vi "XVC_SERVER_UDP.vi"() -> ()   [LabVIEW 2017]
panel:
  out "error out":errorcluster caption="错误输出"
  out "连接的字符串":string
  out "错误输出 5":errorcluster caption="错误输出"
  out "错误输出 4":errorcluster caption="错误输出"
  out "字符串":string
  out "错误输出 3":errorcluster={"status"=TRUE, "code"=56, "source"="TCP Listen.vi:7210001->XVC_SERVER_UDP.vi中的等待TCP侦听器"} caption="错误输出"
  out "错误输出 2":errorcluster={"status"=TRUE, "code"=1, "source"="XVC_SERVER_UDP.vi中的关闭TCP连接"} caption="错误输出"
  out "错误输出":errorcluster
  out "x+1":u32
  in  "data out 5":string="shift:\u0005\u0000\u0000\u0000ÿ\u0000"
  out "received string 2":string
  in  "address":string="192.168.10.20"
  out "received string":string
  out "data out 3":string
  in  "data out 4":string="shift:\u0005\u0000\u0000\u0000ÿ\u0000"
  out "data out 2":string
  out "x != 0?":bool
  in  "Client Closed":string="The client VI closed the connection."
  in  "Stop":bool
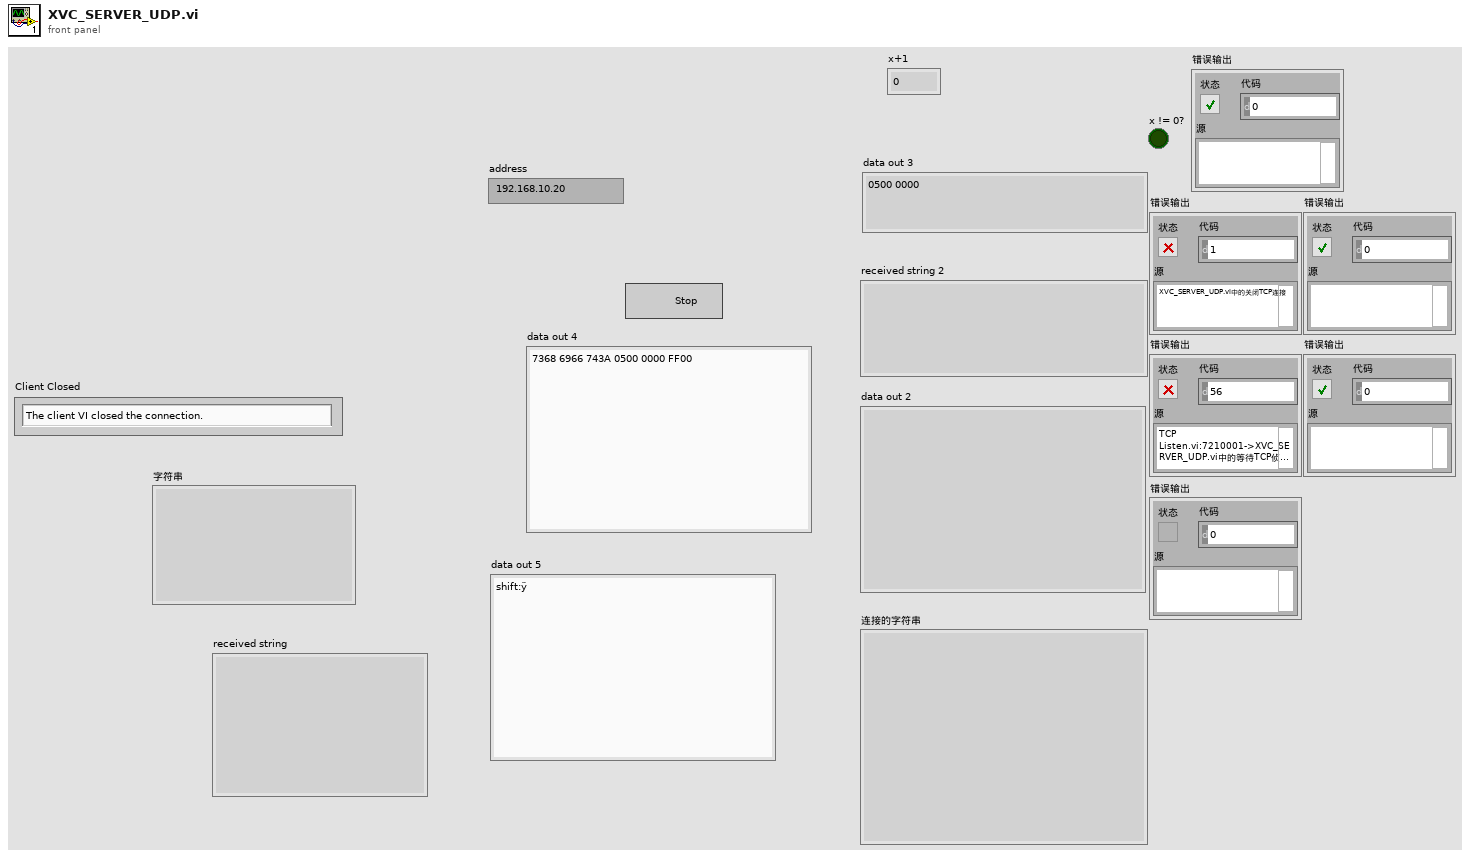
[diagram p1: front panel]
types:
  T1 = enum16{"Standard", "Buffered", "CRLF", "Immediate"}
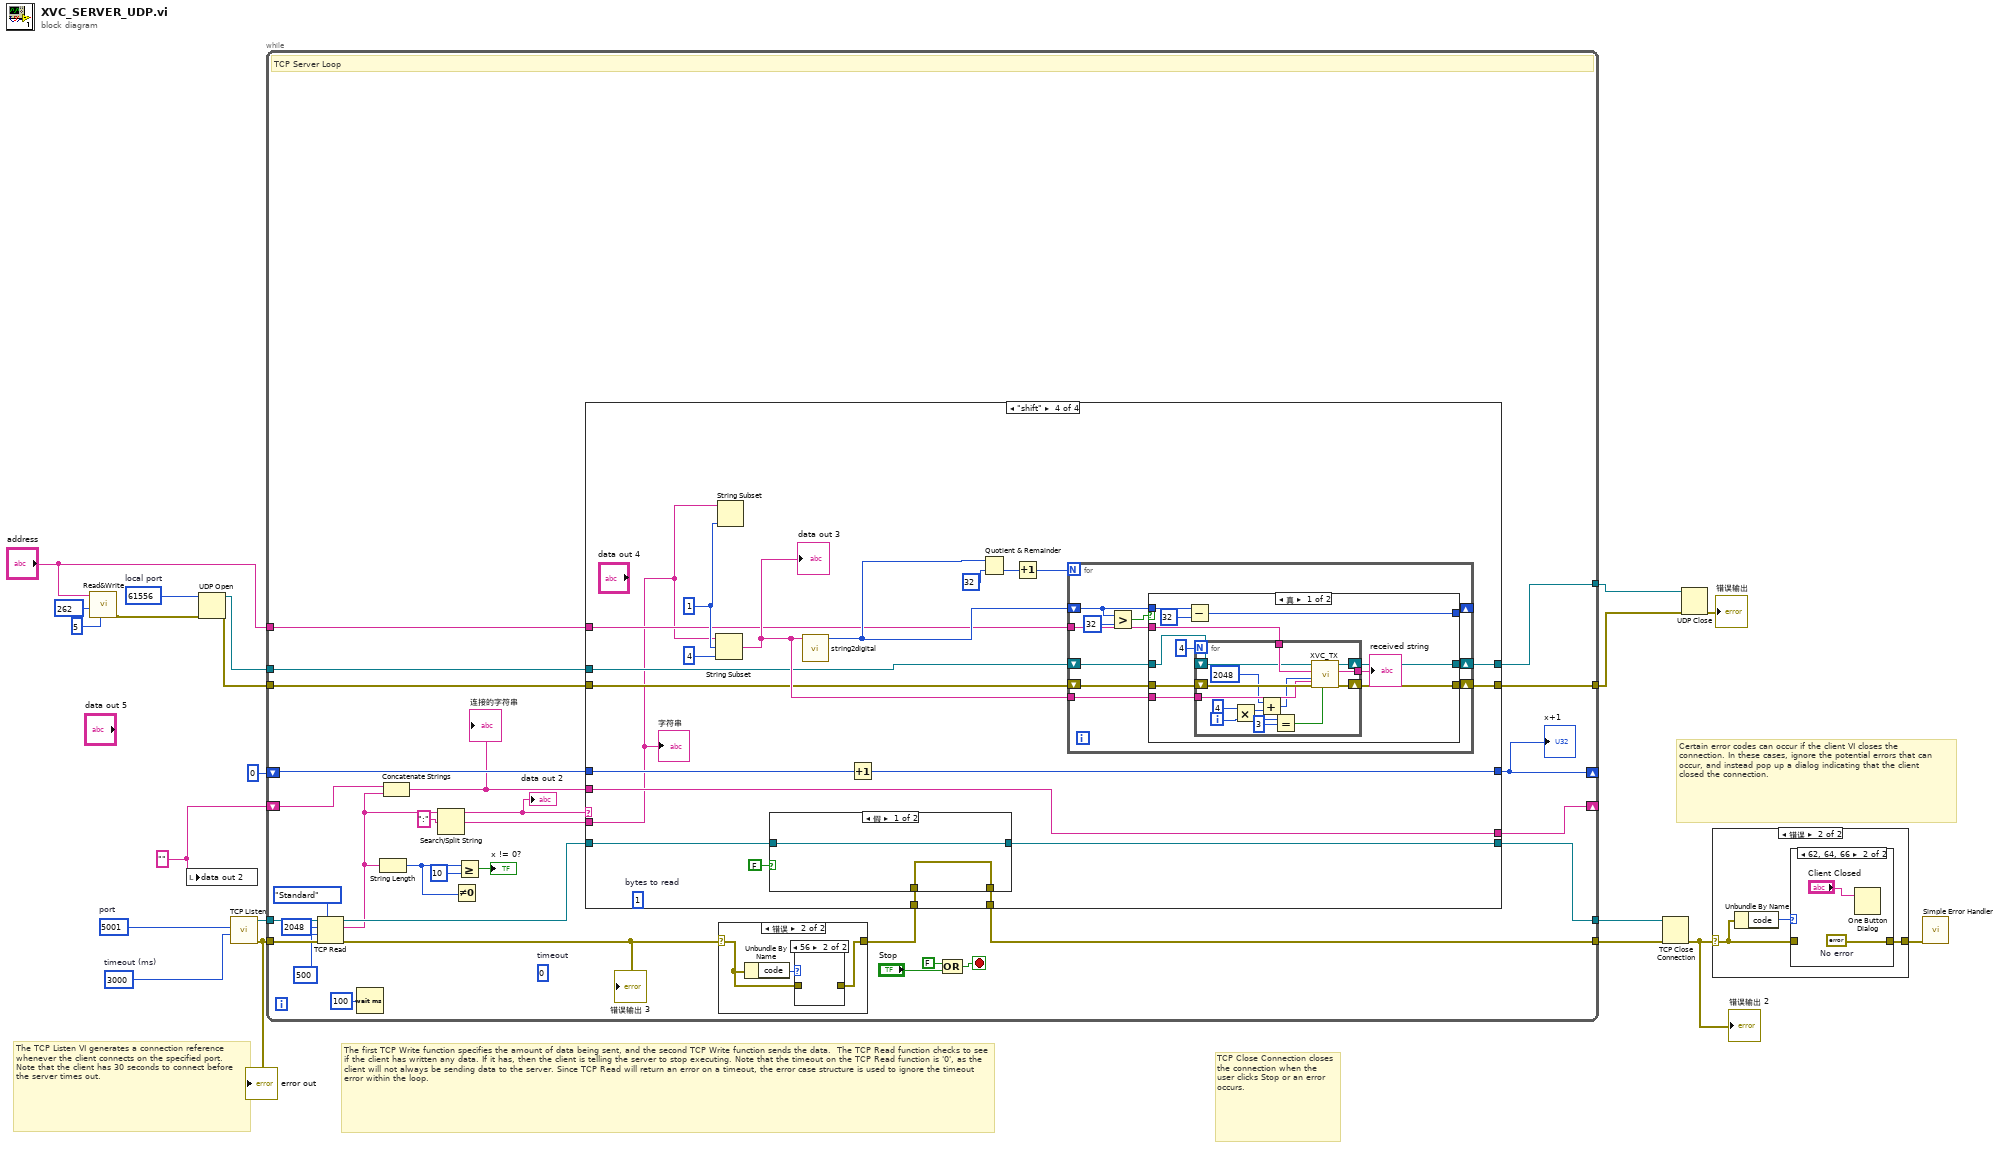
[diagram p0: block diagram]
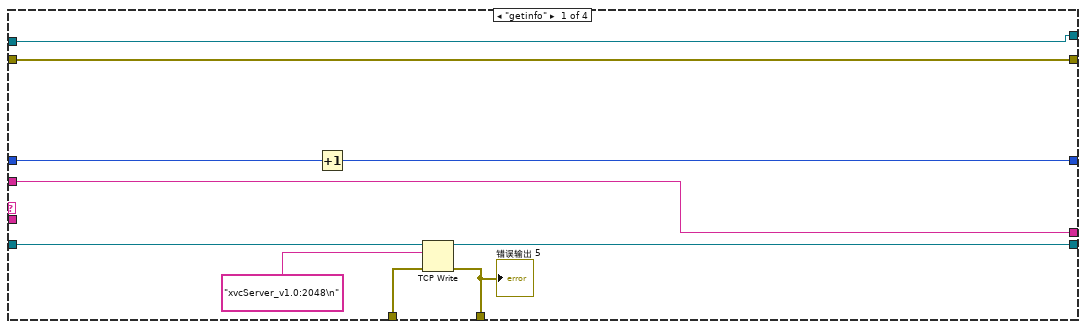
[diagram p4: hidden frame]
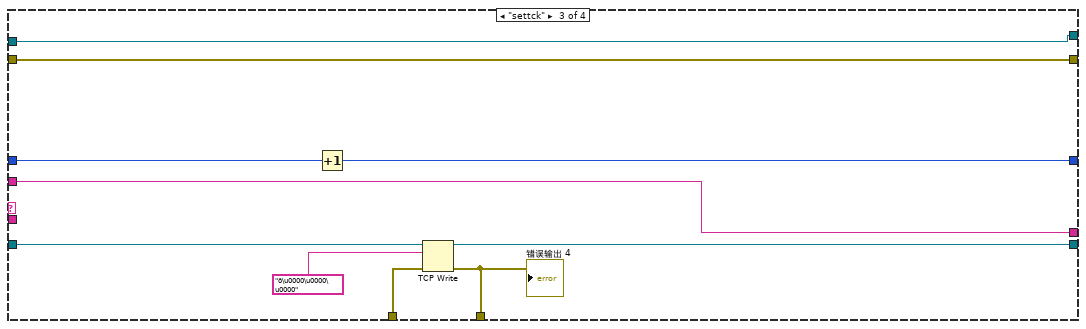
[diagram p6: hidden frame]
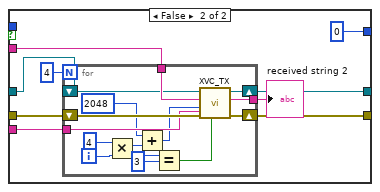
[diagram p7: hidden frame]
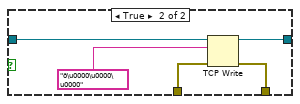
[diagram p8: hidden frame]
diagram:
  w12 = u16 61556  # local port
  w8 = ""
  w13 = u16 5001  # port
  w14 = 3000  # timeout (ms)
  # "TCP Close Connection closes the connection when the user clicks Stop or an error occurs."
  # "The TCP Listen VI generates a connection reference whenever the client connects on the specified port. Note that the client has 30 seconds to connect before the server times out."
  # "Certain error codes can occur if the client VI closes the connection. In these cases, ignore the potential errors that can occur, and instead pop up a dialog indicating that the client closed the connection."
  # "The first TCP Write function specifies the amount of data being sent, and the second TCP Write function sends the data.  The TCP Read function checks to see if the client has written any data. If it has, then the client is telling the server to stop executing. Note that the timeout on the TCP Read function is '0', as the client will not always be sending data to the server. Since TCP Read will return an error on a timeout, the error case structure is used to ignore the timeout error within the loop."
  n1 = call "Read&Write.vi"("In"=u8 5, "Address"=u32 262, "address"="address") -> ("error out"=w9:errorcluster)  [unwired: 7 in, 1 out]
  n2 = local write "data out 2"(w8) -> ()
  n3 = UDP Open(8:w9, 11:w12) -> (port=w4:refnum<k16>, 0:w3:errorcluster)  [unwired: 3 in, 1 out]
  n4 = call <vilib>:"TCP Listen.vi"("timeout ms (wait forever: -1)"=w14, "port"=w13) -> ("error out"=w15:errorcluster, "connection ID"=w16:refnum<k5>)  [unwired: 5 in, 3 out]
  "error out" <- w15
  n5 = while {
    tunnel: [w37] -> w19
    tunnel: [w35] -> w20
    tunnel: w16 -> [w51]
    tunnel: w15 -> [w48]
    shift-right: [w34] -> _
    shift-left: w8 -> [w43]
    shift-right: [w31] -> _
    shift-left: u32 0 -> [w33]
    tunnel: "address" -> [w30]
    tunnel: w4 -> [w29]
    tunnel: w3 -> [w28]
    tunnel: [w27] -> w2
    tunnel: [w26] -> w1
    stop <- w49 stop-if-true
    (unwired) 0  # timeout
    (unwired) 1  # bytes to read
    # "TCP Server Loop"
    n6 = TCP Read(connection ID=w51, bytes to read=2048, error in (no error)=w48, 7:T1."Standard" ("mode (standard)"), 9:500 ("timeout ms (25000)")) -> (connection ID out=w36:refnum<k5>, data out=w25:string, error out=w46:errorcluster)
    "错误输出 3" <- w46
    n7 = Wait (ms)(milliseconds to wait=u32 100) -> ()  [unwired: 1 out]
    n8 = String Length(string=w25) -> (length=w41:i32)
    n9 = Concatenate Strings(w43, w25) -> (w24:string)
    "连接的字符串" <- w24
    n10 = Search/Split String(string=w25, search string/char (-)=":" ("正则表达式")) -> (substring before match=w23:string, match + rest of string=w22:string)  [unwired: 1 in, 1 out]
    "data out 2" <- w23
    n11 = Not Equal To 0?(x=w41) -> ()  [unwired: 1 out]
    n12 = Greater Or Equal?(x=w41, y=10) -> (x >= y?=→"x != 0?":bool)
    n13 = case shown="错误" w46 {
      selector: w46 -> [w164 w166]
      tunnel: [w164 w165] -> w38
      frame No Error {
      }
      frame Error {
        n14 = Unbundle By Name(w166) -> ("code"=w167:i32)
        n15 = case shown="56" w167 {
          tunnel: w166 -> [w168 _]
          tunnel: [w168 _] -> w165
          frame Default {
          }
          frame 56 {
          }
        }
      }
    }
    n16 = case shown="\"shift\"" w23 {
      tunnel: w36 -> [w61 w64 w77 w98]
      tunnel: w38 -> [w59 w63 w75 w97]
      tunnel: [w58 w63 w74 w96] -> w37
      tunnel: [w57 w64 w73 w95] -> w35
      tunnel: [w52 w62 w68 w79] -> w34
      tunnel: [w56 w65 w72 w94] -> w31
      tunnel: w33 -> [w55 w65 w71 w93]
      tunnel: w30 -> [_ _ _ w87]
      tunnel: w29 -> [w54 w67 w70 w86]
      tunnel: w28 -> [w53 w66 w69 w85]
      tunnel: [w53 w66 w69 w84] -> w27
      tunnel: [w54 w67 w70 w83] -> w26
      tunnel: w24 -> [w52 w62 w68 w79]
      tunnel: w22 -> [_ _ _ w78]
      frame "getinfo" {
        n17 = Increment(x=w55) -> (x+1=w56:u32)
        n18 = TCP Write(connection ID=w61, data in="xvcServer_v1.0:2048\n", error in (no error)=w59) -> (connection ID out=w57:refnum<k5>, error out=w58:errorcluster)  [unwired: 1 in, 1 out]
        "错误输出 5" <- w58
      }
      frame "x", Default {
      }
      frame "settck" {
        n19 = Increment(x=w71) -> (x+1=w72:u32)
        n20 = TCP Write(connection ID=w77, data in="ð\u0000\u0000\u0000", error in (no error)=w75) -> (connection ID out=w73:refnum<k5>, error out=w74:errorcluster)  [unwired: 1 in, 1 out]
        "错误输出 4" <- w74
      }
      frame "shift" {
        w88 = 1 ("length (rest)")
        n21 = String Subset(string=w78, offset (0)=w88, length (rest)=4 ("length (rest)")) -> (substring=w90:string)
        "data out 3" <- w90
        n22 = String Subset(string=w78, length (rest)=w88) -> ()  [unwired: 1 in, 1 out]
        n23 = case shown="假" FALSE {
          tunnel: w98 -> [w158 w163]
          tunnel: w97 -> [w157 w161]
          tunnel: [w157 w160] -> w96
          tunnel: [w158 w159] -> w95
          frame False {
          }
          frame True {
            n24 = TCP Write(connection ID=w163, data in="ð\u0000\u0000\u0000", error in (no error)=w161) -> (connection ID out=w159:refnum<k5>, error out=w160:errorcluster)  [unwired: 1 in, 1 out]
          }
        }
        n25 = call "string2digital.vi"("data in"=w90) -> ("number"=w91:u32)  [unwired: 10 in]
        n26 = Increment(x=w93) -> (x+1=w94:u32)
        n27 = Quotient & Remainder(x=w91, y=u8 32) -> (floor(x/y)=w80:u32)  [unwired: 1 out]
        n28 = Increment(x=w80) -> (x+1=w81:u32)
        n29 = for {
          N: w81 -> [_]
          tunnel: w87 -> [w108]
          shift-right: [w106] -> w84
          shift-left: w85 -> [w107]
          shift-right: [w104] -> w83
          shift-left: w86 -> [w105]
          tunnel: w90 -> [w103]
          shift-right: [w99] -> _
          shift-left: w91 -> [w101]
          n30 = Greater?(x=w101, y=u32 32) -> (0:w102:bool)
          n31 = case shown="真" w102 {
            tunnel: w108 -> [w119 w142]
            tunnel: w107 -> [w118 w141]
            tunnel: [w117 w140] -> w106
            tunnel: w105 -> [w116 w139]
            tunnel: [w115 w138] -> w104
            tunnel: w103 -> [w114 w137]
            tunnel: w101 -> [w113 _]
            tunnel: [w111 u32 0] -> w99
            frame True {
              n32 = Subtract(x=w113, y=u32 32) -> (x-y=w111:u32)
              n33 = for {
                N: 4 -> [_]
                tunnel: w119 -> [w133]
                tunnel: w114 -> [w128]
                shift-right: [w131] -> w117
                shift-left: w118 -> [w132]
                shift-right: [w129] -> w115
                shift-left: w116 -> [w130]
                tunnel: [w120] -> w109
                i -> [w123]
                n34 = Multiply(x=4, y=w123) -> (x*y=w126:i32)
                n35 = Add(x=u32 2048 ("Address"), y=w126) -> (x+y=w124:u32)
                n36 = Equal?(x=w123, y=3) -> (x = y?=w121:bool)
                n37 = call "XVC_TX.vi"("data in"=w128, "Read (TRUE)"=w121, "error in"=w132, "Address"=w124, "IP address"=w133, "connection ID"=w130) -> ("error out"=w131:errorcluster, "received string"=w120:string, "connection ID 2"=w129:refnum<k16>)  [unwired: 3 in]
              }
              "received string" <- w109
            }
            frame False {
              n38 = for {
                N: 4 -> [_]
                tunnel: w142 -> [w156]
                tunnel: w137 -> [w151]
                shift-right: [w154] -> w140
                shift-left: w141 -> [w155]
                shift-right: [w152] -> w138
                shift-left: w139 -> [w153]
                tunnel: [w143] -> w135
                i -> [w146]
                n39 = Multiply(x=4, y=w146) -> (x*y=w149:i32)
                n40 = Add(x=u32 2048 ("Address"), y=w149) -> (x+y=w147:u32)
                n41 = Equal?(x=w146, y=3) -> (x = y?=w144:bool)
                n42 = call "XVC_TX.vi"("data in"=w151, "Read (TRUE)"=w144, "error in"=w155, "Address"=w147, "IP address"=w156, "connection ID"=w153) -> ("error out"=w154:errorcluster, "received string"=w143:string, "connection ID 2"=w152:refnum<k16>)  [unwired: 3 in]
              }
              "received string 2" <- w135
            }
          }
        }
        "字符串" <- w78
      }
    }
    "x+1" <- w31
    n43 = Compound Arithmetic op=OR(FALSE ("值"), "Stop") -> (w49:bool)
  }
  n44 = TCP Close Connection(connection ID=w20, error in (no error)=w19) -> (error out=w18:errorcluster)  [unwired: 2 out]
  "错误输出 2" <- w18
  n45 = UDP Close(connection ID=w1, 8:w2) -> (error out=→"错误输出":errorcluster)  [unwired: 1 out]
  n46 = case shown="错误" w18 {
    selector: w18 -> [w169 w171]
    tunnel: [w169 w170] -> w17
    frame No Error {
    }
    frame Error {
      n47 = Unbundle By Name(w171) -> ("code"=w172:i32)
      n48 = case shown="62, 64, 66" w172 {
        tunnel: w171 -> [w173 _]
        tunnel: [w173 w175] -> w170
        frame Default {
        }
        frame 62, 64, 66 {
          w175 = errorcluster {"status"=FALSE, "code"=0, "source"=""}  # No error
          n49 = One Button Dialog(message="Client Closed") -> ()  [unwired: 1 in, 1 out]
        }
      }
    }
  }
  n50 = call <vilib>:"Simple Error Handler.vi"("error in (no error)"=w17) -> ()  [unwired: 1 in, 8 out]
